vi "Test PC Unlocker.vi"   [LabVIEW 2016, in "Script.lvlib"]
uses:
  Script.lvlib
  <vilib>/SLL Drona/APIs/Stimulus/KeyBoardSimulation/typedef/Action.ctl
  <vilib>/SLL Drona/APIs/Stimulus/KeyBoardSimulation/typedef/VirtualKey.ctl
  <vilib>/Wiresmith Technology/G CLI/Argument Parser/Option Class/Argument Type.ctl
  <vilib>/Wiresmith Technology/G CLI/Argument Parser/Option Class/Option.lvclass
  <vilib>/Wiresmith Technology/G CLI/Argument Parser/Option Class/Option Configuration.ctl
  <vilib>/SLL Drona/APIs/Stimulus/KeyBoardSimulation/KeyboardSimulationCore.vi
types:
  T1 = typedef "Option Parser.lvlib/Option.lvclass/Option Configuration.ctl" = cluster{"Option Type":T2, "Option Labels":string[], "Key":string, "Description":string, "Required":bool, "Default Value":string}
  T2 = typedef "Option Parser.lvlib/Option.lvclass/Argument Type.ctl" = enum16{"flag", "value"}
  T3 = typedef "Drona.lvlib/KeyboardSimulation.lvlib/VirtualKey.ctl" = u8
  T4 = typedef "Drona.lvlib/KeyboardSimulation.lvlib/Action.ctl" = enum16{"Press", "Up", "Down"}
  T5 = cluster{"Key":T3, "Action":T4, "Delay (ms)":u32}[]
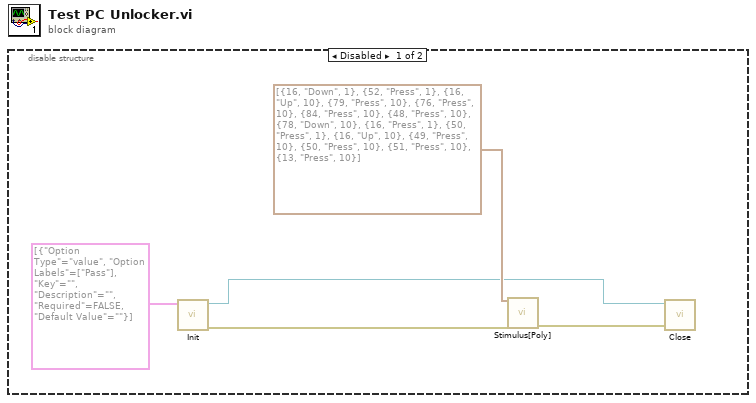
[diagram p0: block diagram]
diagram:
  n1 = disable-structure shown="Disabled" {
    frame Disabled {
      n2 = call "Init.vi"("Options"=T1[] [{"Option Type"=enum."value", "Option Labels"=["Pass"], "Key"="", "Description"="", "Required"=FALSE, "Default Value"=""}]) -> ("error out"=w3:errorcluster, "CLI out"=w2:refnum<class "CLI.lvclass">)  [unwired: 8 in, 1 out]
      n3 = call-poly <vilib>:"Stimulus[Poly].vi"("Key Array"=T5 [{"Key"=16, "Action"=enum."Down", "Delay (ms)"=1}, {"Key"=52, "Action"=enum."Press", "Delay (ms)"=1}, {"Key"=16, "Action"=enum."Up", "Delay (ms)"=10}, {"Key"=79, "Action"=enum."Press", "Delay (ms)"=10}, {"Key"=76, "Action"=enum."Press", "Delay (ms)"=10}, {"Key"=84, "Action"=enum."Press", "Delay (ms)"=10}, {"Key"=48, "Action"=enum."Press", "Delay (ms)"=10}, {"Key"=78, "Action"=enum."Down", "Delay (ms)"=10}, {"Key"=16, "Action"=enum."Press", "Delay (ms)"=1}, {"Key"=50, "Action"=enum."Press", "Delay (ms)"=1}, {"Key"=16, "Action"=enum."Up", "Delay (ms)"=10}, {"Key"=49, "Action"=enum."Press", "Delay (ms)"=10}, {"Key"=50, "Action"=enum."Press", "Delay (ms)"=10}, {"Key"=51, "Action"=enum."Press", "Delay (ms)"=10}, {"Key"=13, "Action"=enum."Press", "Delay (ms)"=10}], "error in"=w3) -> ("error out"=w1:errorcluster)  [unwired: 13 in]
      n4 = call "Close.vi"("error in (no error)"=w1, "CLI in"=w2) -> ()  [unwired: 10 in]
    }
    frame Enabled {
    }
  }
